vi "Write ScaleAndLimitConfig.vi"(8 "error in (no error)":errorcluster, 10 "ScaleAndLimitConfig":T1[](array[typedef]), 11 "ScaleAndLimitModule configuration in":refnum<class "ScaleAndLimitModule configuration.lvclass">) -> (0 "error out":errorcluster, 3 "ScaleAndLimitModule configuration out":refnum<class "ScaleAndLimitModule configuration.lvclass">)   [LabVIEW 2017, in "ScaleAndLimitModule configuration.lvclass"]
uses:
  ScaleAndLimitModule configuration.lvclass
  <vilib>/NI/PowerElectronicsControl/ScaleAndLimit/Interface/Configuration.ctl
  ScaleAndLimitModule configuration.lvclass/ScaleAndLimitModule configuration.ctl
  <vilib>/NI/PowerElectronicsControl/ScaleAndLimit/Interface/ScaleAndLimitInterface.lvlib
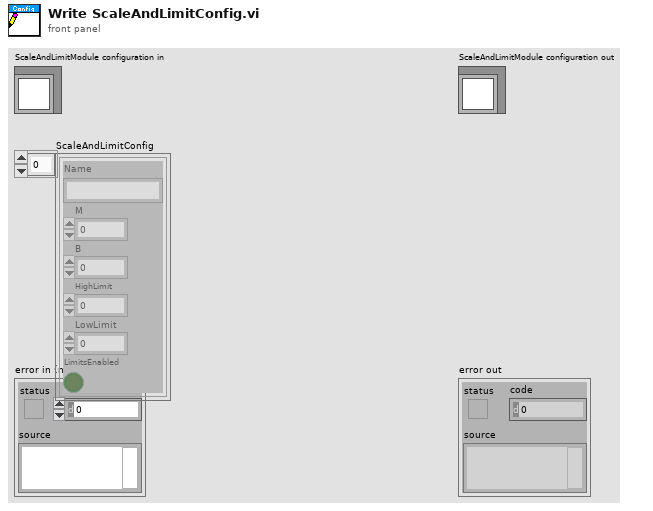
[diagram p1: front panel]
types:
  T1 = typedef "ScaleAndLimitInterface.lvlib/Configuration.ctl" = cluster{"Name":string, "M":dbl, "B":i16, "HighLimit":dbl, "LowLimit":dbl, "LimitsEnabled":bool}
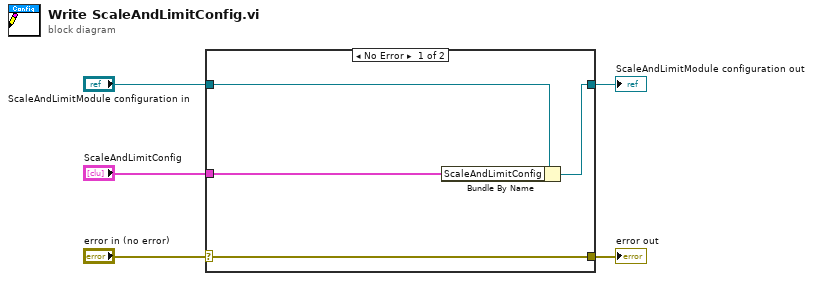
[diagram p0: block diagram]
diagram:
  n1 = case shown="No Error" "error in (no error)" {
    selector: "error in (no error)" -> [w9 w10]
    tunnel: [w9 w10] -> w4
    tunnel: [w7 w11] -> w2
    tunnel: "ScaleAndLimitModule configuration in" -> [w8 w11]
    tunnel: "ScaleAndLimitConfig" -> [w6 _]
    frame No Error {
      n2 = Bundle By Name(cluster=w8, "ScaleAndLimitConfig"=w6) -> (w7:refnum<class "ScaleAndLimitModule configuration.lvclass">)
    }
    frame Error {
    }
  }
  "error out" <- w4
  "ScaleAndLimitModule configuration out" <- w2
